vi "ControlExists.vi"(10 "ControlName":string, 11 "ControlsPath":path) -> (2 "Boolean":bool, 3 "ControlPath":path)   [LabVIEW 2015]
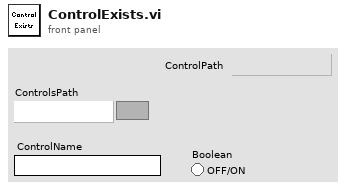
[diagram p1: front panel]
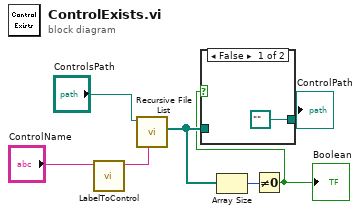
[diagram p0: block diagram]
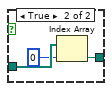
[diagram p2: hidden frame]
diagram:
  n1 = call "LabelToControl.vi"("ControlName"="ControlName") -> ("String"=w5:string)  [unwired: 10 in]
  n2 = call <vilib>:"Recursive File List.vi"("pattern"=w5, "Folder Path"="ControlsPath") -> ("All Files in Dir"=w3:path[])  [unwired: 5 in, 4 out]
  n3 = Array Size(array=w3) -> (size(s)=w7:i32)
  n4 = Not Equal To 0?(x=w7) -> (x != 0?=w1:bool)
  "Boolean" <- w1
  n5 = case shown="False" w1 {
    tunnel: w3 -> [_ w11]
    tunnel: [path "" w9] -> w2
    frame False {
    }
    frame True {
      n6 = Index Array(array=w11, index=0) -> (element=w9:path)
    }
  }
  "ControlPath" <- w2
